vi "BuildTemplatePadLists.vi"() -> (1 "RealTime":string[](array[string]), 2 "Templates":string[](array[string]), 3 "ScratchPads":string[](array[string]), 5 "All Templates":string[](array[string]))   [LabVIEW 2022 SP3]
uses:
  Mic/Mic_Global.vi
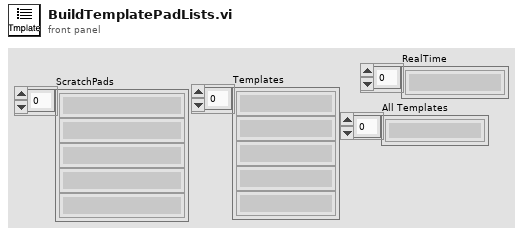
[diagram p1: front panel]
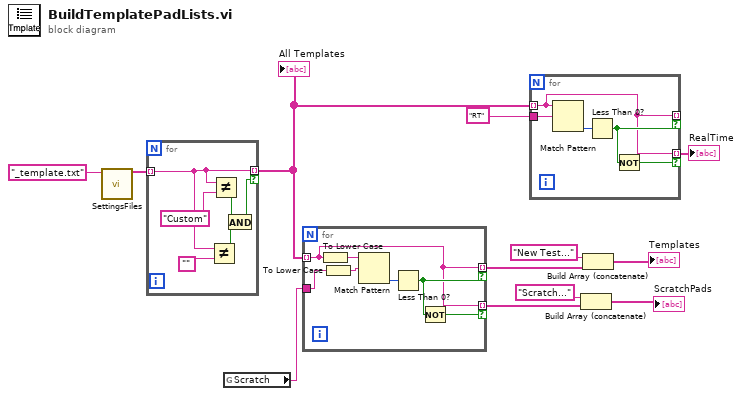
[diagram p0: block diagram]
diagram:
  n1 = call "SettingsFiles.vi"("settings file name"="_template.txt" ("pattern")) -> ("filenames"=w1:string[])  [unwired: 9 in, 1 out]
  n2 = for {
    tunnel: w1 -> [w13] mode=indexing
    tunnel: [w13] -> w3 mode=indexing if=w14
    n3 = Not Equal?(x=w13, y="") -> (x != y?=w16:bool)
    n4 = Not Equal?(x=w13, y="Custom") -> (x != y?=w15:bool)
    n5 = And(x=w15, y=w16) -> (x .and. y?=w14:bool)
  }
  "All Templates" <- w3
  n6 = global read "Mic_Global.vi" "Scratch"() -> (w11:string)
  n7 = for {
    tunnel: w3 -> [w21] mode=indexing
    tunnel: w11 -> [w25]
    tunnel: [w21] -> w5 mode=indexing if=w23
    tunnel: [w21] -> w9 mode=indexing if=w22
    n8 = To Lower Case(string=w21) -> (all lower case string=w20:string)
    n9 = To Lower Case(string=w25) -> (all lower case string=w19:string)
    n10 = Match Pattern(string=w20, regular expression=w19) -> (offset past match=w24:i32)  [unwired: 4 out]
    n11 = Less Than 0?(x=w24) -> (x < 0?=w23:bool)
    n12 = Not(x=w23) -> (.not. x?=w22:bool)
  }
  n13 = for {
    tunnel: w3 -> [w26] mode=indexing
    tunnel: "RT" ("regular expression") -> [w30]
    tunnel: [w26] -> _ mode=indexing if=w28
    tunnel: [w26] -> w10 mode=indexing if=w27
    n14 = Match Pattern(string=w26, regular expression=w30) -> (offset past match=w29:i32)  [unwired: 4 out]
    n15 = Less Than 0?(x=w29) -> (x < 0?=w28:bool)
    n16 = Not(x=w28) -> (.not. x?=w27:bool)
  }
  "RealTime" <- w10
  n17 = Build Array (concatenate)("Scratch..." ("y"), w9) -> (→"ScratchPads":string[])
  n18 = Build Array (concatenate)("New Test..." ("y"), w5) -> (→"Templates":string[])
